vi "cburen_Chrg_Dschrg.vi"(4 "PS VISA in":refnum<visa-resource-name>, 5 "PS error in":errorcluster, 6 "DischargeCyclePath":path=path "C:/Users/ga11/Desktop/VI/results/3PtestCharge.lvm" caption="Filename", 8 "Charge/discharge":enum8{"Charge", "Discharge"}(ring), 9 "Charge/Discharge Voltage Setpoint":dbl format="%#.6g", 10 "CC or CCCV":enum16{"CC", "CCCV"}(ring), 11 "Current Setpoint":dbl format="%#.6g", 12 "Output Safety":T1, 13 "Current Cutoff":dbl) -> (18 "PS VIS resource name out":refnum<visa-resource-name>, 19 "PS error out":errorcluster)   [LabVIEW 2020]
uses:
  Battery-Testing-Software-NHR/system_development/v0.1/Drivers-NHR-9200/NHR/Public/Data/Read (Ave Current).vi
  Battery-Testing-Software-NHR/system_development/v0.1/Drivers-NHR-9200/NHR/Public/Data/Low Level/Fetch (Ave Voltage).vi
  Battery-Testing-Software-NHR/system_development/v0.1/Drivers-Essentials/NH Research Regenerative Test Series.lvlib
panel:
  out "Read Ave Current (A)":dbl
  out "Read Ave Voltage (V)":dbl
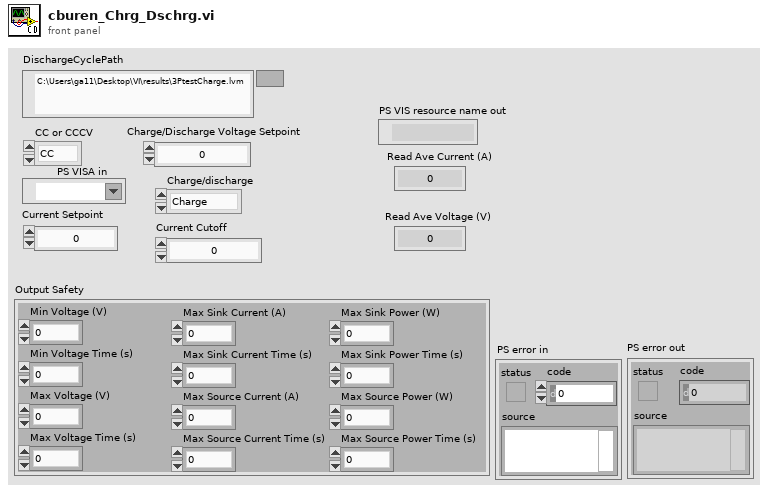
[diagram p1: front panel]
types:
  T1 = cluster{"Min Voltage (V)":dbl, "Min Voltage Time (s)":dbl, "Max Voltage (V)":dbl, "Max Voltage Time (s)":dbl, "Max Sink Current (A)":dbl, "Max Sink Current Time (s)":dbl, "Max Source Current (A)":dbl, "Max Source Current Time (s)":dbl, "Max Sink Power (W)":dbl, "Max Sink Power Time (s)":dbl, "Max Source Power (W)":dbl, "Max Source Power Time (s)":dbl}
  T2 = cluster{"Voltage Enabled":bool, "Current Enabled":bool, "Power Enabled":bool, "Resistance Enabled":bool}
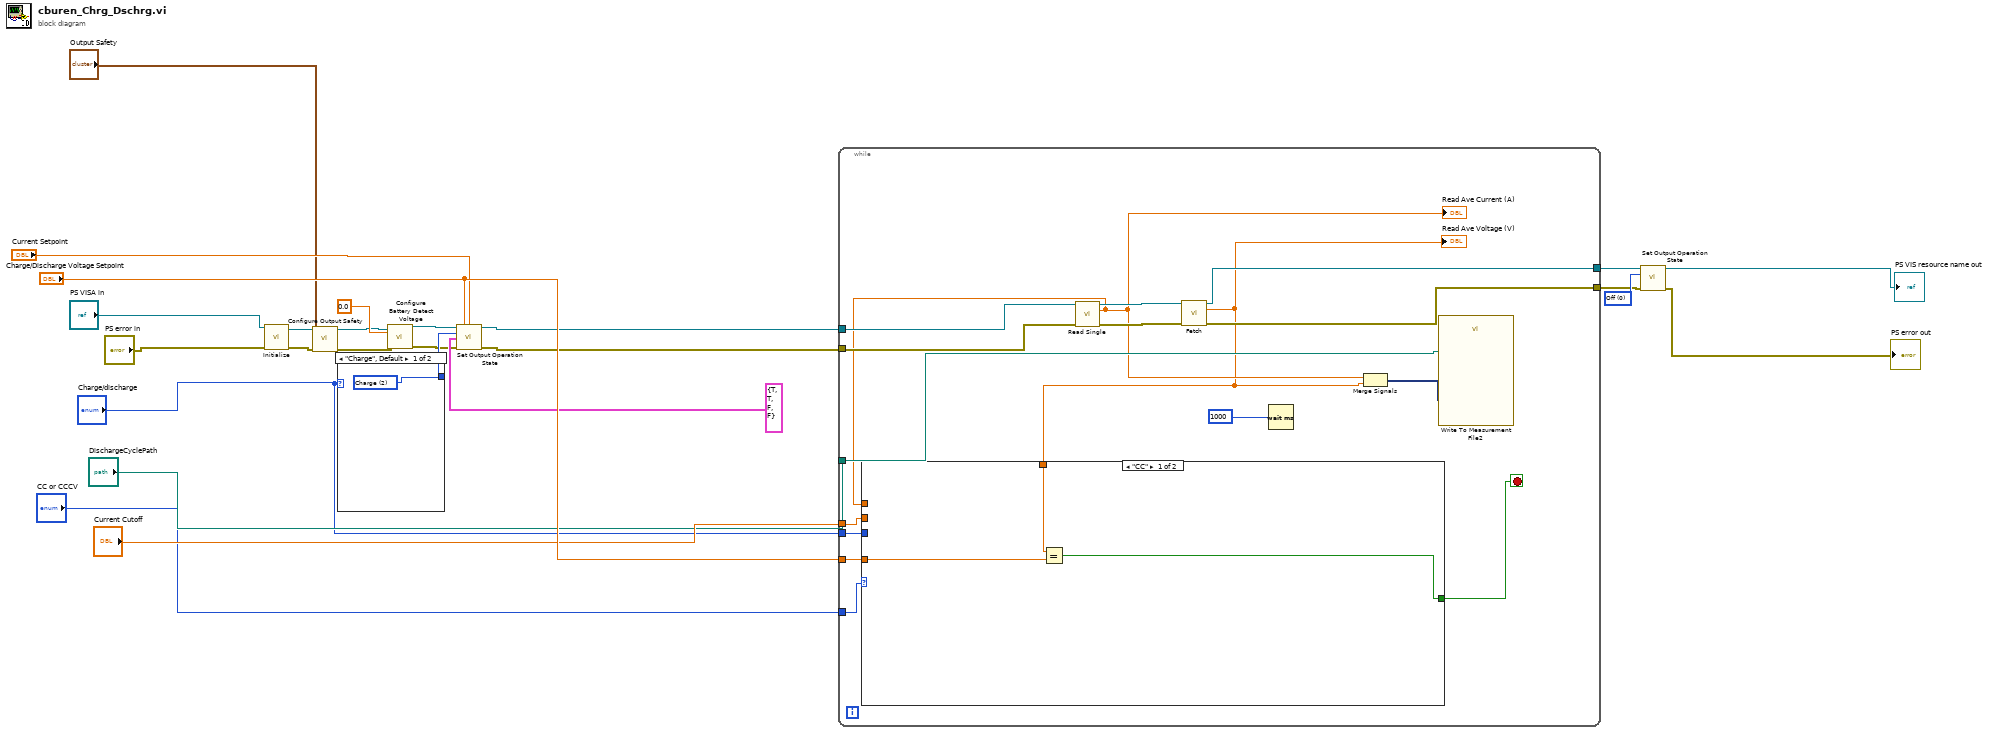
[diagram p0: block diagram]
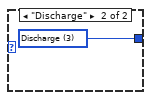
[diagram p2: hidden frame]
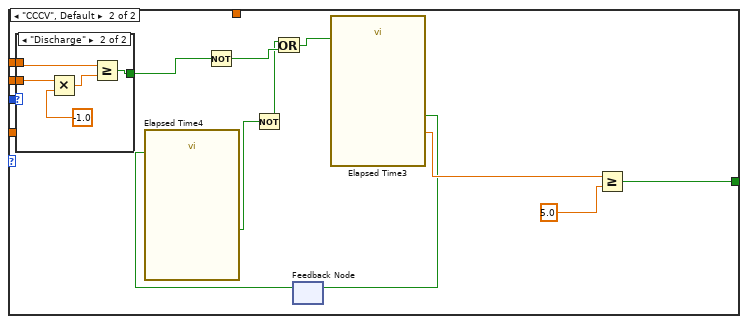
[diagram p3: hidden frame]
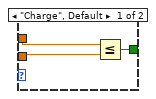
[diagram p4: hidden frame]
diagram:
  w13 = 0 items=["Off", "Standby", "Charge", "Discharge", "Battery"] ("Mode (0: Off)")
  n1 = call "Initialize.vi"("VISA resource name"="PS VISA in", "error in (no error)"="PS error in") -> ("VISA resource name out"=w4:refnum<visa-resource-name>, "error out"=w5:errorcluster)  [unwired: 12 in]
  n2 = call "Configure Output Safety.vi"("VISA resource name"=w4, "Output Safety"="Output Safety", "error in (no error)"=w5) -> ("VISA resource name out"=w7:refnum<visa-resource-name>, "error out"=w6:errorcluster)  [unwired: 11 in]
  n3 = case shown="\"Charge\", Default" "Charge/discharge" {
    tunnel: [w26 w27] -> w14
    frame "Charge", Default {
      w26 = 2 items=["Off", "Standby", "Charge", "Discharge", "Battery"] ("Mode (0: Off)")
    }
    frame "Discharge" {
      w27 = 3 items=["Off", "Standby", "Charge", "Discharge", "Battery"] ("Mode (0: Off)")
    }
  }
  n4 = call "Configure Battery Detect Voltage.vi"("VISA resource name"=w7, "Battery Detect Voltage (0V)"=0.0, "error in (no error)"=w6) -> ("VISA resource name out"=w12:refnum<visa-resource-name>, "error out"=w11:errorcluster)  [unwired: 11 in]
  n5 = call "Set Output Operation State.vi"("VISA resource name"=w12, "Voltage Setpoint (0 V)"="Charge/Discharge Voltage Setpoint", "Current Setpoint (0 A)"="Current Setpoint", "Mode (0: Off)"=w14, "Enable"=T2 {"Voltage Enabled"=TRUE, "Current Enabled"=TRUE, "Power Enabled"=FALSE, "Resistance Enabled"=FALSE}, "error in (no error)"=w11) -> ("VISA resource name out"=w17:refnum<visa-resource-name>, "error out"=w16:errorcluster)  [unwired: 8 in]
  n6 = while {
    tunnel: w17 -> [w41]
    tunnel: w16 -> [w40]
    tunnel: "Current Cutoff" -> [w33]
    tunnel: "DischargeCyclePath" -> [w36]
    tunnel: [w35] -> w9
    tunnel: [w34] -> w8
    tunnel: "CC or CCCV" -> [w31]
    tunnel: "Charge/Discharge Voltage Setpoint" -> [w30]
    tunnel: "Charge/discharge" -> [w29]
    stop <- w37 stop-if-true
    n7 = call-poly "Read Single.vi"("VISA resource name"=w41, "error in (no error)"=w40) -> ("VISA resource name out"=w42:refnum<visa-resource-name>, "Ave Current (A)"=w32:dbl, "error out"=w43:errorcluster)  [unwired: 11 in]
    "Read Ave Current (A)" <- w32
    n8 = call-poly "Fetch.vi"("VISA resource name"=w42, "error in (no error)"=w43) -> ("VISA resource name out"=w35:refnum<visa-resource-name>, "Ave Voltage (V)"=w28:dbl, "error out"=w34:errorcluster)  [unwired: 11 in]
    "Read Ave Voltage (V)" <- w28
    n9 = case shown="\"CC\"" w31 {
      tunnel: [w44 w53] -> w37
      tunnel: w33 -> [_ w50]
      tunnel: w32 -> [_ w49]
      tunnel: w28 -> [w46 _]
      tunnel: w30 -> [w45 _]
      tunnel: w29 -> [_ w47]
      frame "CC" {
        n10 = Equal?(x=w46, y=w45) -> (x = y?=w44:bool)
      }
      frame "CCCV", Default {
        n11 = case shown="\"Discharge\"" w47 {
          tunnel: w50 -> [w61 w66]
          tunnel: w49 -> [w62 w64]
          tunnel: [w60 w63] -> w48
          frame "Charge", Default {
            n12 = Less Or Equal?(x=w62, y=w61) -> (x <= y?=w60:bool)
          }
          frame "Discharge" {
            n13 = Multiply(x=w66, y=-1.0) -> (x*y=w65:dbl)
            n14 = Greater Or Equal?(x=w64, y=w65) -> (x >= y?=w63:bool)
          }
        }
        n15 = Not(x=w48) -> (.not. x?=w59:bool)
        n16 = feedback #1() -> (w51:bool)  [unwired: 1 in]
        n17 = call "Elapsed Time4"("Reset"=w51) -> ("Time has Elapsed"=w58:bool)  [unwired: 11 in, 7 out]
        n18 = Not(x=w58) -> (.not. x?=w57:bool)
        n19 = Or(x=w57, y=w59) -> (x .or. y?=w56:bool)
        n20 = call "Elapsed Time3"("Reset"=w56) -> ("Elapsed Time (s)"=w55:dbl, "Time has Elapsed"=w52:bool)  [unwired: 11 in, 6 out]
        n21 = feedback-in #1(w52) -> ()
        n22 = Greater Or Equal?(x=w55, y=5.0) -> (x >= y?=w53:bool)
      }
    }
    n23 = Wait (ms)(milliseconds to wait=1000) -> ()  [unwired: 1 out]
    n24 = Merge Signals "Merge Signals"(w32, w28) -> (w39:dynamicdata)
    n25 = call "Write To Measurement File2"("Signals"=w39, "Filename"=w36) -> ()  [unwired: 15 in, 3 out]
  }
  n26 = call "Set Output Operation State.vi"("VISA resource name"=w9, "Mode (0: Off)"=w13, "error in (no error)"=w8) -> ("VISA resource name out"=→"PS VIS resource name out":refnum<visa-resource-name>, "error out"=→"PS error out":errorcluster)  [unwired: 11 in]
